vi "BARCODE SCAN 710N  KEYANCE.vi"(1 "byte count":u32=24, 11 "VISA resource name":refnum<visa-resource-name>) -> (3 "leak":string)   [LabVIEW 2015]
uses:
  <vilib>/Instr/_visa.llb/VISA Configure Serial Port (Instr).vi
  Variable/Global.vi
panel:
  out "OK":bool
  out "Stoped":bool
  in  "Stoped 2":bool
  out "array":string[](array[string])
  out "read string":string
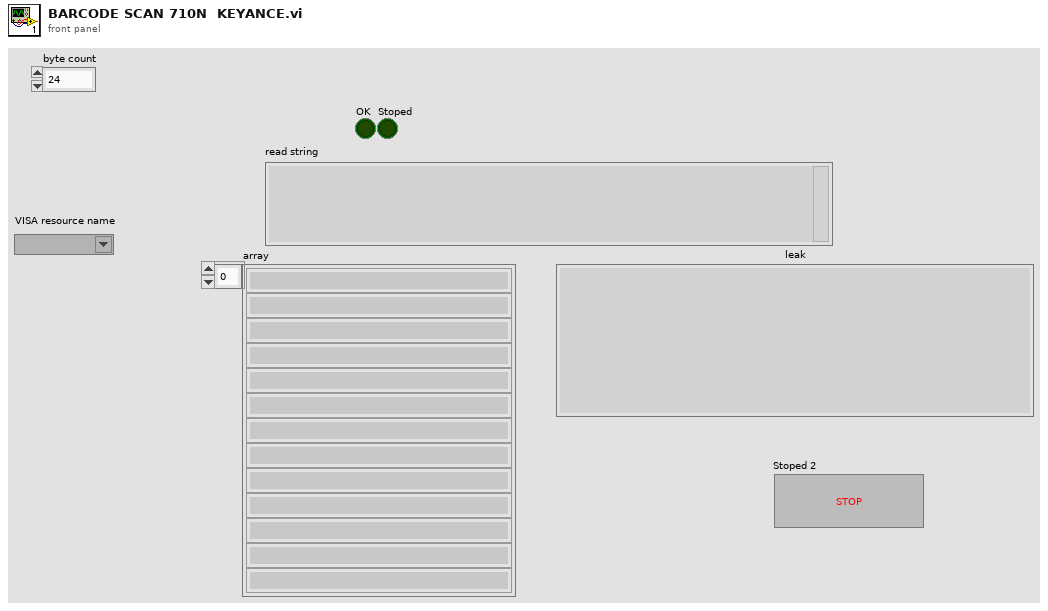
[diagram p1: front panel]
types:
  T1 = cluster{"Barcode Scanner 2":refnum<visa-resource-name>, "baud rate":u32, "data bits":u16, "parity":enum16{"None", "Odd", "Even", "Mark", "Space"}, "stop bits":u16, "flow control":u16}
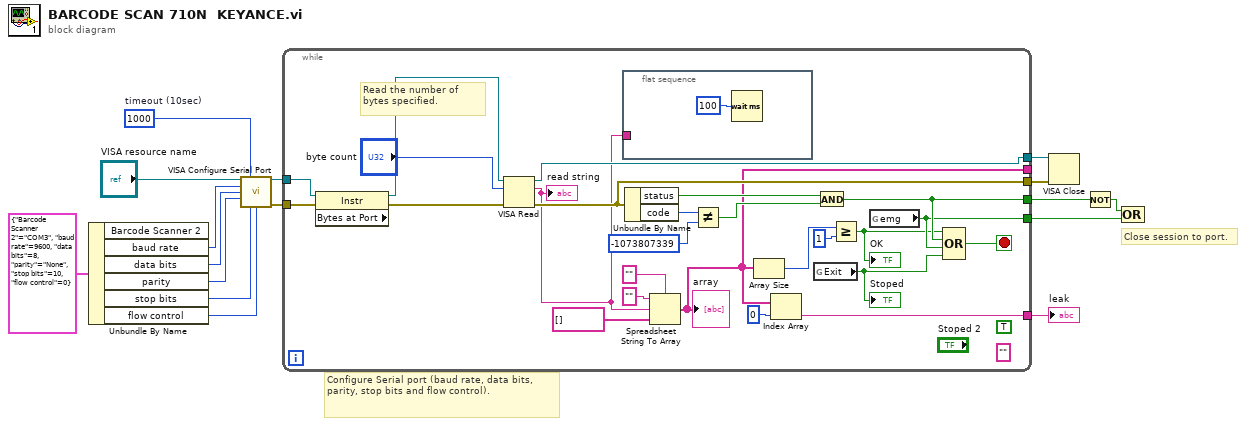
[diagram p0: block diagram]
diagram:
  w9 = u32 1000  # timeout (10sec)
  # "Close session to port."
  # "Configure Serial port (baud rate, data bits, parity, stop bits and flow control)."
  n1 = Unbundle By Name(T1 {"Barcode Scanner 2"="COM3", "baud rate"=9600, "data bits"=8, "parity"=enum."None", "stop bits"=10, "flow control"=0} ("Serial Parameters")) -> ("baud rate"=w11:u32, "data bits"=w12:u16, "parity"=w13:enum16{"None", "Odd", "Even", "Mark", "Space"}, "stop bits"=w14:u16, "flow control"=w15:u16)  [unwired: 1 out]
  n2 = call-poly "VISA Configure Serial Port"("VISA resource name"="VISA resource name", "timeout (10sec)"=w9, "baud rate (9600)"=w11, "data bits (8)"=w12, "parity (0:none)"=w13, "stop bits (10: 1 bit)"=w14, "flow control (0:none)"=w15) -> ("VISA resource name out"=w8:refnum<visa-resource-name>, "error out"=w7:errorcluster)  [unwired: 2 in, 5 out]
  n3 = while {
    tunnel: [w40] -> w6
    tunnel: [w41] -> w5
    tunnel: w7 -> [w26]
    tunnel: w8 -> [w29]
    tunnel: [w34] -> w4
    tunnel: [w20] -> w3
    tunnel: [w22] -> _
    tunnel: [w21] -> w1
    stop <- w39 stop-if-true
    (unwired) ""
    (unwired) TRUE ("OK")
    # "Read the number of bytes specified."
    n4 = property class="Instr" props=["Bytes at Port"](reference=w29, error in=w26) -> (reference out=w28:refnum<visa-resource-name>, error out=w27:errorcluster)  [unwired: 1 out]
    n5 = VISA Read(VISA resource name=w28, byte count="byte count", error in (no error)=w27) -> (VISA resource name out=w41:refnum<visa-resource-name>, read buffer=w23:string, error out=w40:errorcluster)  [unwired: 1 out]
    "read string" <- w23
    n6 = flat-sequence {
      tunnel: w23 -> [_]
      frame #0 {
        n7 = Wait (ms)(milliseconds to wait=u32 100) -> ()  [unwired: 1 out]
      }
    }
    n8 = Unbundle By Name(w40) -> ("status"=w38:bool, "code"=w37:i32)
    n9 = Spreadsheet String To Array(delimiter (Tab)="", format string="", spreadsheet string=w23, array type (2D Dbl)=string[] []) -> (array=w22:string[])
    "array" <- w22
    n10 = Not Equal?(x=w37, y=-1073807339 ("code")) -> (x != y?=w35:bool)
    n11 = Array Size(array=w22) -> (size(s)=w25:i32)
    n12 = Index Array(array=w22, index=0) -> (element=w21:string)
    n13 = global read "Global.vi" "Exit"() -> (w19:bool)
    "Stoped" <- w19
    n14 = And(x=w38, y=w35) -> (x .and. y?=w34:bool)
    n15 = Greater Or Equal?(x=w25, y=1) -> (x >= y?=w18:bool)
    "OK" <- w18
    n16 = global read "Global.vi" "emg"() -> (w20:bool)
    n17 = Compound Arithmetic op=OR(w18, w34, w20, w19) -> (w39:bool)
  }
  "leak" <- w1
  n18 = VISA Close(VISA resource name=w5, error in (no error)=w6) -> ()  [unwired: 1 out]
  n19 = Not(x=w4) -> (.not. x?=w2:bool)
  n20 = Compound Arithmetic op=OR(w2, w3) -> ()  [unwired: 1 out]
